vi "system_identification.vi"() -> ()   [LabVIEW 2020]
uses:
  <vilib>/ptbypt/NI_PtbyPt.lvlib
panel:
  out "LSE1,LSE2":cluster{dbl, dbl}(graph)
  in  "standard deviation":dbl=1.0 format="%0.2f"
  out "LMS Filter 2":dbl[](array[numeric])
  out "LMS Filter 1":dbl[](array[numeric])
  out "Error e[n] 2":dbl(graph)
  out "Error e[n] 1":dbl(graph)
  in  "Adaptive Filter Length":i32
  in  "milliseconds to wait":u32
  in  "FIR Filter Coefficients":dbl[](array[numeric])
  in  "stop":bool
  in  "LMS Filter2 Step Size, mu":dbl
  in  "LMS Filter1 Step Size, mu":dbl
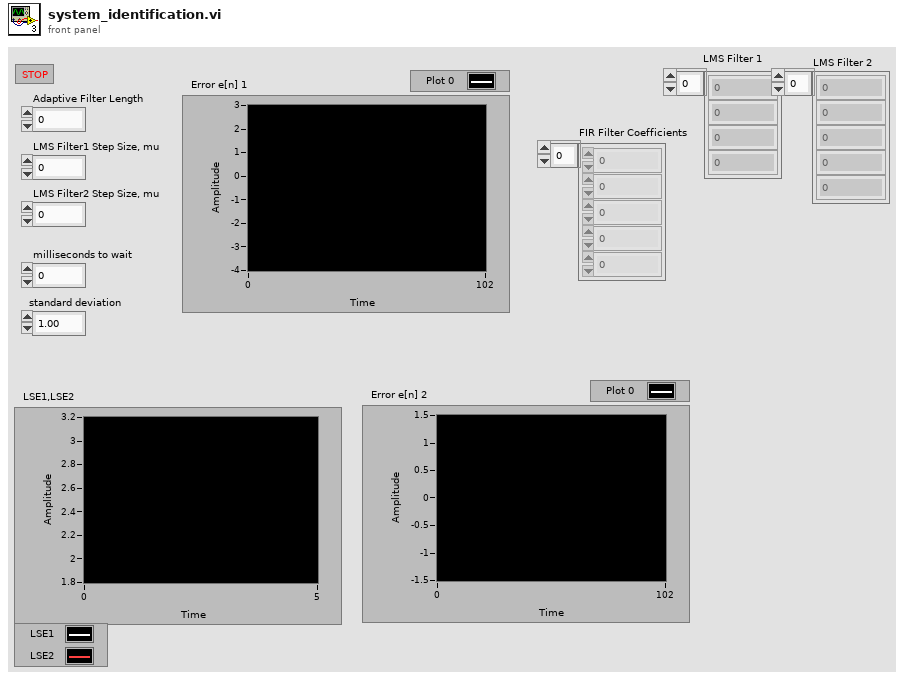
[diagram p1: front panel]
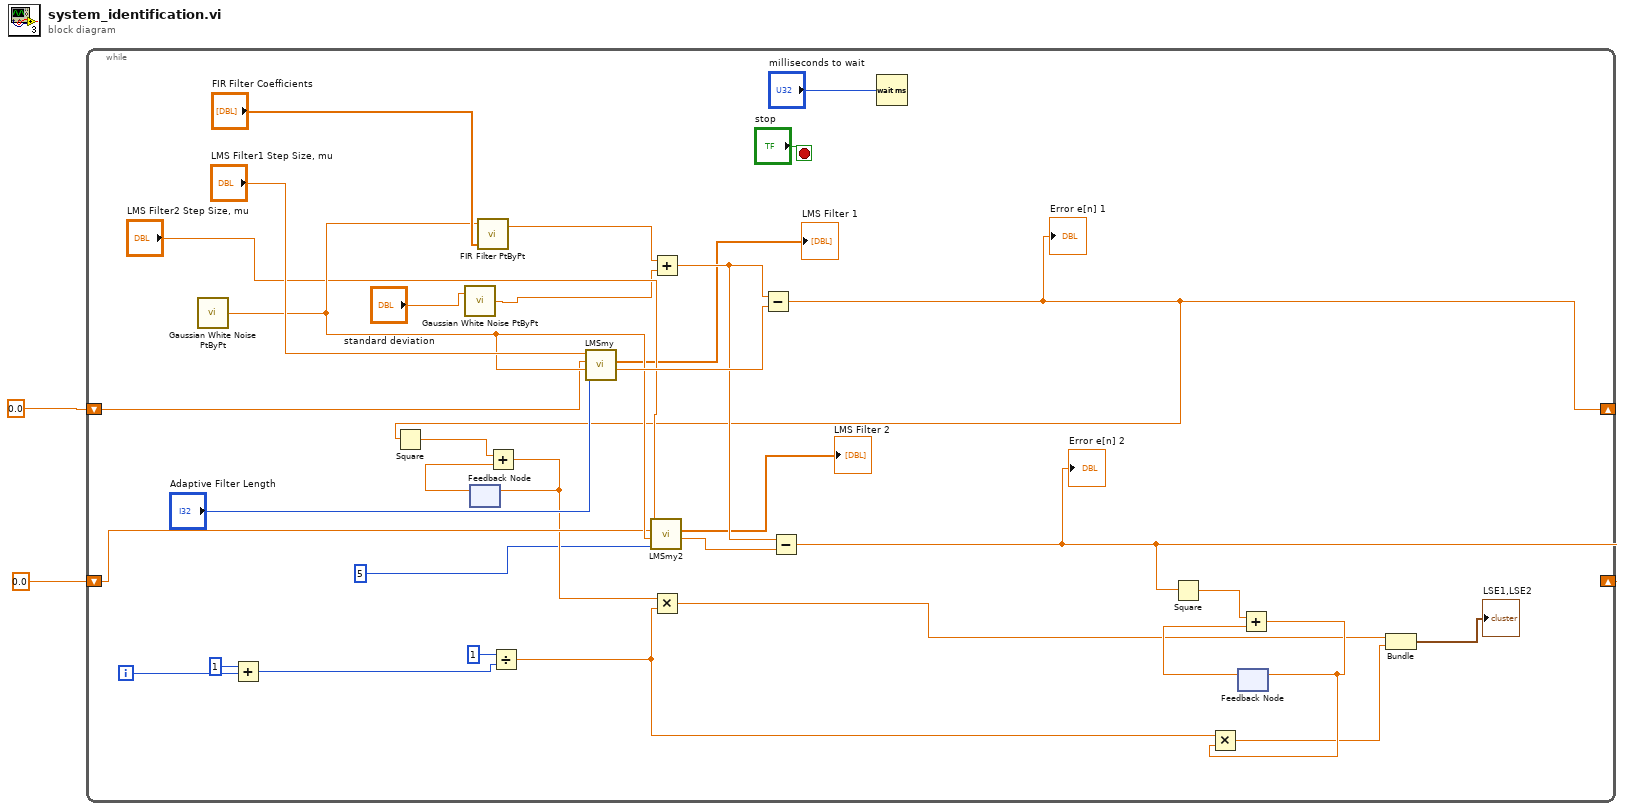
[diagram p0: block diagram]
diagram:
  n1 = while {
    shift-right: [w14] -> _
    shift-left: 0.0 -> [w18]
    shift-right: [w21] -> _
    shift-left: 0.0 -> [w29]
    i -> [w5]
    stop <- "stop" stop-if-true
    n2 = call <vilib>:"Gaussian White Noise PtByPt.vi"() -> ("Gaussian white noise"=w30:dbl)  [unwired: 3 in]
    n3 = Add(x=1, y=w5) -> (x+y=w19:i32)
    n4 = call <vilib>:"Gaussian White Noise PtByPt.vi"("standard deviation"="standard deviation") -> ("Gaussian white noise"=w3:dbl)  [unwired: 2 in]
    n5 = feedback #1() -> (w16:dbl)  [unwired: 1 in]
    n6 = call <vilib>:"FIR Filter PtByPt.vi"("Forward Coefficients"="FIR Filter Coefficients", "x"=w30) -> ("Filtered x"=w33:dbl)  [unwired: 2 in, 1 out]
    n7 = Divide(x=1, y=w19) -> (x/y=w11:dbl)
    n8 = call "LMSmy.vi"("sample length"="Adaptive Filter Length", "x(n+1) input point"=w30, "error e(n)"=w18, "mu"="LMS Filter1 Step Size, mu") -> ("y(n+1)"=w32:dbl, "w(n)"=→"LMS Filter 1":dbl[])  [unwired: 6 in]
    n9 = call "LMSmy2.vi"("sample length"=5, "x(n+1) input point"=w30, "error e(n)"=w29, "mu"="LMS Filter2 Step Size, mu") -> ("y(n+1)"=w27:dbl, "w(n)"=→"LMS Filter 2":dbl[])  [unwired: 6 in]
    n10 = Add(x=w33, y=w3) -> (x+y=w28:dbl)
    n11 = Subtract(x=w28, y=w32) -> (x-y=w14:dbl)
    "Error e[n] 1" <- w14
    n12 = Square(x=w14) -> (x^2=w17:dbl)
    n13 = Add(x=w17, y=w16) -> (x+y=w15:dbl)
    n14 = feedback-in #1(w15) -> ()
    n15 = Multiply(x=w15, y=w11) -> (x*y=w9:dbl)
    n16 = Subtract(x=w28, y=w27) -> (x-y=w21:dbl)
    "Error e[n] 2" <- w21
    n17 = Wait (ms)(milliseconds to wait="milliseconds to wait") -> ()  [unwired: 1 out]
    n18 = Square(x=w21) -> (x^2=w13:dbl)
    n19 = feedback #2() -> (w12:dbl)  [unwired: 1 in]
    n20 = Add(x=w13, y=w12) -> (x+y=w10:dbl)
    n21 = Multiply(x=w11, y=w10) -> (x*y=w8:dbl)
    n22 = feedback-in #2(w10) -> ()
    n23 = Bundle(w9, w8) -> (→"LSE1,LSE2":cluster{dbl, dbl})  [unwired: 1 in]
  }
